vi "Initialize.vi"(5 "TCP Configuration":T1, 7 "Serial Port":refnum<visa-resource-name>="COM13", 8 "Error In":errorcluster, 10 "Interface":T2, 11 "Platform":T8) -> (0 "Error Out":errorcluster={"status"=FALSE, "code"=1073676294, "source"="VISA Read in LVH-LINX.lvlib:Device.lvlib:Serial Read.vi->LVH-LINX.lvlib:Device.lvlib:Wait For Packet.vi->LVH-LINX.lvlib:Device.lvlib:Send Command.vi->LVH-LINX.lvlib:Device.lvlib:Get DIO Channels.vi->LVH-LINX.lvlib:Device.lvlib:Load Device Config.vi->LVH-LINX.lvlib:Device.lvlib:Initialize Device.vi->LVH-LINX.lvlib:Initialize.vi->Untitled 2"}, 2 "Device Name":string, 3 "LINX Ref":T3={"Platform"=enum."LINX", "Interface"=enum."Serial", "LINX Device Config"={"Interface"=enum."Serial", "COM Port"="COM13", "TCP Configuration"={"IP Address"="", "Port"=0}, "Device Family"=enum."Digilent", "Device ID"=1, "Device Name"="myRIO-1900", "TCP Ref"=refnum, "Channels"={"DI Channels"=[0, 1, 2, 3, 4, 5, 6, 7, 8, 9, 10, 11, 12, 13, 14, 15, 16, 17, 18, 19, 20, 21, 22, 23, 24, 25, 26, 27, 28, 29, 30, 31, 32, 33, 34, 35, 36, 37, 38, 39, 40, 41, 42, 43, 44, 45, 46], "DO Channels"=[0, 1, 2, 3, 4, 5, 6, 7, 8, 9, 10, 11, 12, 13, 14, 15, 16, 17, 18, 19, 20, 21, 22, 23, 24, 25, 26, 27, 28, 29, 30, 31, 32, 33, 34, 35, 36, 37, 38, 39, 40, 41, 42, 43, 44, 45, 46], "AI"=[0, 1, 2, 3, 4, 5, 6, 7, 8, 9, 10, 11], "AO"=[], "PWM"=[3, 5, 6, 9, 10], "QE"=[], "UART"=[0, 1], "I2C 2"=[0], "SPI"=[0], "CAN"=[], "AI Ref (V)"=3.3, "AO Resolution (Bits)"=0, "AO Ref (V)"=0.0}}})   [LabVIEW 2013, in "LVH-LINX.lvlib"]
doc: "Initialize a connection to a LINX device."
uses:
  LVH-LINX.lvlib
  Private/Type Defs/User Platform.ctl
  Private/Type Defs/LINX Ref.ctl
  Private/Type Defs/Platform.ctl
  Private/Type Defs/Interface.ctl
  Private/Device/Type Defs/LINX Device Config.ctl
  Private/Device/Type Defs/TCP Config.ctl
  Private/Type Defs/Device Family.ctl
  Private/Device/Type Defs/Channels.ctl
  Private/Type Defs/Channel FGV States.ctl
  Private/Device/Device.lvlib
  Private/Type Defs/Devices - NI.ctl
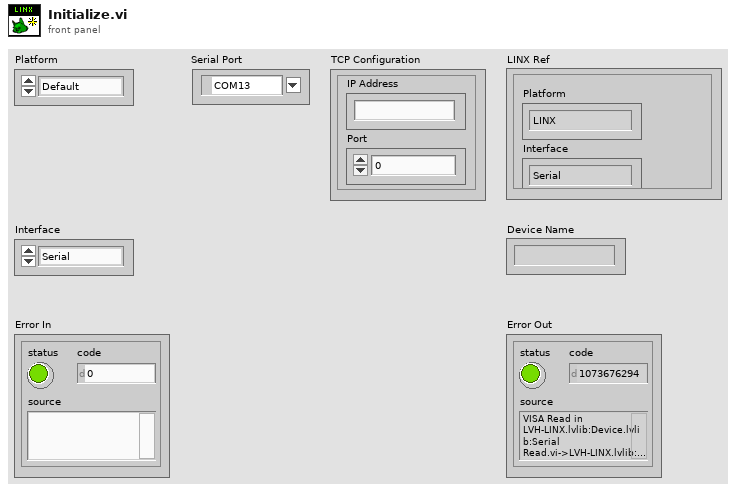
[diagram p1: front panel]
types:
  T1 = typedef "LVH-LINX.lvlib/Device.lvlib/TCP Config.ctl" = cluster{"IP Address":string, "Port":u16}
  T2 = typedef "LVH-LINX.lvlib/Interface.ctl" = enum16{"Serial", "TCP"}
  T3 = typedef "LVH-LINX.lvlib/LINX Ref.ctl" = cluster{"Platform":T4, "Interface":T2, "LINX Device Config":T5}
  T4 = typedef "LVH-LINX.lvlib/Platform.ctl" = enum16{"LINX", "myRIO"}
  T5 = typedef "LVH-LINX.lvlib/Device.lvlib/LINX Device Config.ctl" = cluster{"Interface":T2, "COM Port":refnum<visa-resource-name>, "TCP Configuration":T1, "Device Family":T6, "Device ID":u8, "Device Name":string, "TCP Ref":refnum<k5>, "Channels":T7}
  T6 = typedef "LVH-LINX.lvlib/Device Family.ctl" = enum8{"National Instruments", "Digilent", "Arduino"}
  T7 = typedef "LVH-LINX.lvlib/Channels.ctl" = cluster{"DI Channels":u8[], "DO Channels":u8[], "AI":u8[], "AO":u8[], "PWM":u8[], "QE":u8[], "UART":u8[], "I2C 2":u8[], "SPI":u8[], "CAN":u8[], "AI Ref (V)":dbl, "AO Resolution (Bits)":u8, "AO Ref (V)":dbl}
  T8 = typedef "LVH-LINX.lvlib/User Platform.ctl" = enum16{"Default", "LINX", "myRIO"}
  T9 = typedef "LVH-LINX.lvlib/Devices - NI.ctl" = enum16{"myRIO-1900", "myRIO-1950"}
  T10 = typedef "LVH-LINX.lvlib/Channel FGV States.ctl" = enum16{"Initialize", "Get", "Set"}
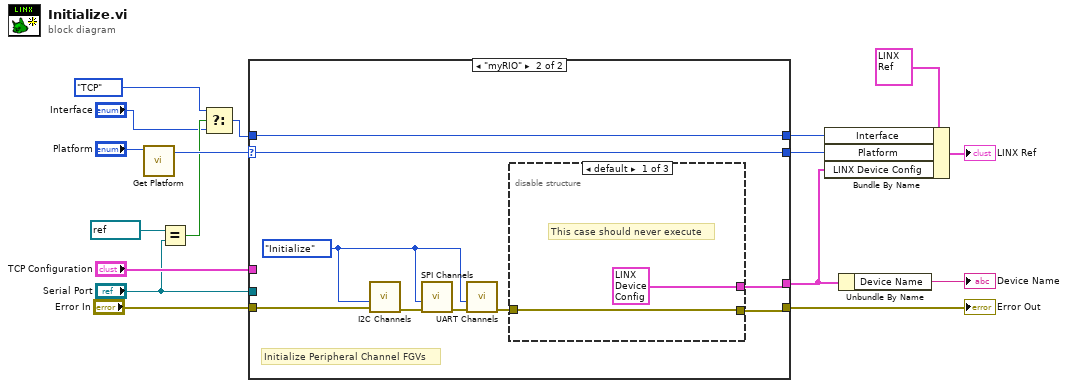
[diagram p0: block diagram]
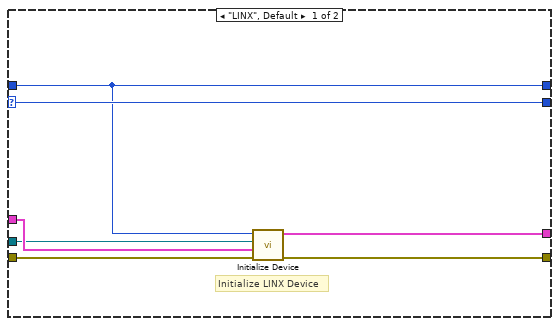
[diagram p2: hidden frame]
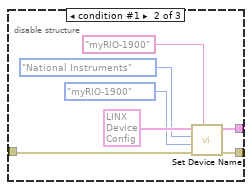
[diagram p3: hidden frame]
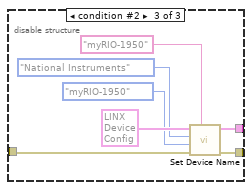
[diagram p4: hidden frame]
diagram:
  n1 = call "Get Platform.vi"("Platform"="Platform") -> ("Platform"=w15:T4)  [unwired: 10 in]
  n2 = Equal?(x=refnum<visa-resource-name> "N/A", y="Serial Port") -> (x = y?=w4:bool)
  n3 = Select(t=Interface."TCP" ("f"), s=w4, f="Interface") -> (s? t:f=w3:T2)
  n4 = case shown="\"myRIO\"" w15 {
    selector: w15 -> [w24 w33]
    tunnel: [w21 w30] -> w8
    tunnel: [w22 w29] -> w13
    tunnel: "Error In" -> [w23 w31]
    tunnel: [w24 w33] -> w10
    tunnel: "Serial Port" -> [w19 _]
    tunnel: w3 -> [w18 w32]
    tunnel: "TCP Configuration" -> [w20 _]
    tunnel: [w18 w32] -> w9
    frame "LINX", Default {
      # "Initialize LINX Device"
      n5 = call "Initialize Device.vi"("Error In"=w23, "TCP Configuration"=w20, "COM Port"=w19, "Interface"=w18) -> ("Error Out"=w22:errorcluster, "LINX Device Config"=w21:T5)  [unwired: 6 in]
    }
    frame "myRIO" {
      w25 = Channel_FGV_States."Initialize" ("Channel State")
      # "Initialize Peripheral Channel FGVs"
      n6 = call "I2C Channels.vi"("Error In"=w31, "Channel State"=w25) -> ("Error Out"=w28:errorcluster)  [unwired: 8 in, 1 out]
      n7 = call "SPI Channels.vi"("Error In"=w28, "Channel State"=w25) -> ("Error Out"=w27:errorcluster)  [unwired: 8 in, 1 out]
      n8 = call "UART Channels.vi"("Error In"=w27, "Channel State"=w25) -> ("Error Out"=w26:errorcluster)  [unwired: 8 in, 1 out]
      n9 = disable-structure shown="default" {
        disable-tunnel: w26 -> [w35 w40 w43]
        disable-tunnel: [T5 {"Interface"=enum."Serial", "COM Port"="", "TCP Configuration"={"IP Address"="", "Port"=0}, "Device Family"=enum."National Instruments", "Device ID"=0, "Device Name"="", "TCP Ref"=refnum, "Channels"={"DI Channels"=[], "DO Channels"=[], "AI"=[], "AO"=[], "PWM"=[], "QE"=[], "UART"=[], "I2C 2"=[], "SPI"=[], "CAN"=[], "AI Ref (V)"=0.0, "AO Resolution (Bits)"=0, "AO Ref (V)"=0.0}} ("LINX Device Config") w42 w45] -> w30
        disable-tunnel: [w35 w41 w44] -> w29
        frame condition #0 (active) {
          # "This case should never execute"
        }
        frame condition #1 {
          n10 = call <vilib>:"Set Device Name.vi"("Device Name"="myRIO-1900", "Error In"=w40, "Device ID"=Devices_-_NI."myRIO-1900" ("NI Device"), "Device Family"=Device_Family."National Instruments", "LINX Device Config"=T5 {"Interface"=enum."Serial", "COM Port"="", "TCP Configuration"={"IP Address"="", "Port"=0}, "Device Family"=enum."National Instruments", "Device ID"=0, "Device Name"="", "TCP Ref"=refnum, "Channels"={"DI Channels"=[], "DO Channels"=[], "AI"=[], "AO"=[], "PWM"=[], "QE"=[], "UART"=[], "I2C 2"=[], "SPI"=[], "CAN"=[], "AI Ref (V)"=0.0, "AO Resolution (Bits)"=0, "AO Ref (V)"=0.0}}) -> ("Error Out"=w41:errorcluster, "LINX Device Config"=w42:T5)  [unwired: 5 in]
        }
        frame condition #2 {
          n11 = call <vilib>:"Set Device Name.vi"("Device Name"="myRIO-1950", "Error In"=w43, "Device ID"=Devices_-_NI."myRIO-1950" ("NI Device"), "Device Family"=Device_Family."National Instruments", "LINX Device Config"=T5 {"Interface"=enum."Serial", "COM Port"="", "TCP Configuration"={"IP Address"="", "Port"=0}, "Device Family"=enum."National Instruments", "Device ID"=0, "Device Name"="", "TCP Ref"=refnum, "Channels"={"DI Channels"=[], "DO Channels"=[], "AI"=[], "AO"=[], "PWM"=[], "QE"=[], "UART"=[], "I2C 2"=[], "SPI"=[], "CAN"=[], "AI Ref (V)"=0.0, "AO Resolution (Bits)"=0, "AO Ref (V)"=0.0}}) -> ("Error Out"=w44:errorcluster, "LINX Device Config"=w45:T5)  [unwired: 5 in]
        }
      }
    }
  }
  "Error Out" <- w13
  n12 = Bundle By Name(cluster=T3 {"Platform"=enum."LINX", "Interface"=enum."Serial", "LINX Device Config"={"Interface"=enum."Serial", "COM Port"="", "TCP Configuration"={"IP Address"="", "Port"=0}, "Device Family"=enum."National Instruments", "Device ID"=0, "Device Name"="", "TCP Ref"=refnum, "Channels"={"DI Channels"=[], "DO Channels"=[], "AI"=[], "AO"=[], "PWM"=[], "QE"=[], "UART"=[], "I2C 2"=[], "SPI"=[], "CAN"=[], "AI Ref (V)"=0.0, "AO Resolution (Bits)"=0, "AO Ref (V)"=0.0}}} ("LINX Resource"), "Interface"=w9, "Platform"=w10, "LINX Device Config"=w8) -> (→"LINX Ref":T3)
  n13 = Unbundle By Name(w8) -> ("Device Name"=→"Device Name":string)
